vi "Adler32.vi"(11 "input_string":string="hello world") -> (3 "Adler32":u32)   [LabVIEW 2020]
panel:
  # "An implementation of the Adler32 checksum,\nsee https://en.wikipedia.org/wiki/Adler-32\nand https://tools.ietf.org/html/rfc1950"
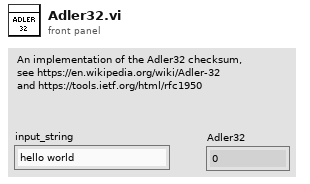
[diagram p1: front panel]
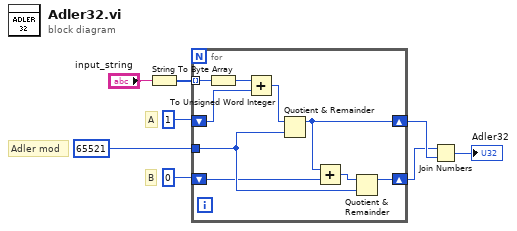
[diagram p0: block diagram]
diagram:
  # "B"
  # "A"
  # "Adler mod"
  n1 = String To Byte Array(string="input_string") -> (unsigned byte array=w4:u8[])
  n2 = for {
    shift-right: [w9] -> w3
    shift-left: u16 1 ("s1") -> [w16]
    shift-right: [w10] -> w2
    shift-left: u16 0 ("s1") -> [w14]
    tunnel: u16 65521 -> [w17]
    tunnel: w4 -> [w12] mode=indexing
    n3 = To Unsigned Word Integer(number=w12) -> (unsigned 16bit integer=w11:u16)
    n4 = Add(x=w11, y=w16) -> (x+y=w15:u16)
    n5 = Quotient & Remainder(x=w15, y=w17) -> (x-y*floor(x/y)=w9:u16)  [unwired: 1 out]
    n6 = Add(x=w9, y=w14) -> (x+y=w13:u16)
    n7 = Quotient & Remainder(x=w13, y=w17) -> (x-y*floor(x/y)=w10:u16)  [unwired: 1 out]
  }
  n8 = Join Numbers(hi=w2, lo=w3) -> ((hi.lo)=→"Adler32":u32)
